vi "Get Ctl Value.vi"(8 "error in (no error)":errorcluster, 10 "Control Refs":refnum<vi>[](array[refnum]), 11 "Part in":refnum<class "Part.lvclass">) -> (0 "error out":errorcluster, 3 "Part out":refnum<class "Part.lvclass">)   [LabVIEW 2015, in "Part.lvclass"]
uses:
  Part.lvclass
  Part.lvclass/Part.ctl
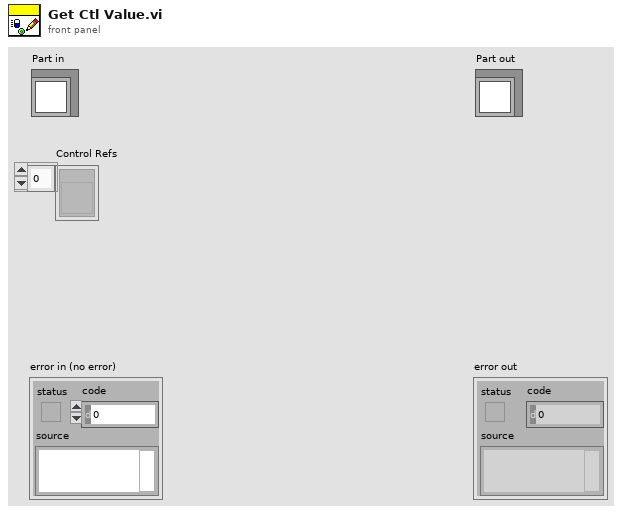
[diagram p1: front panel]
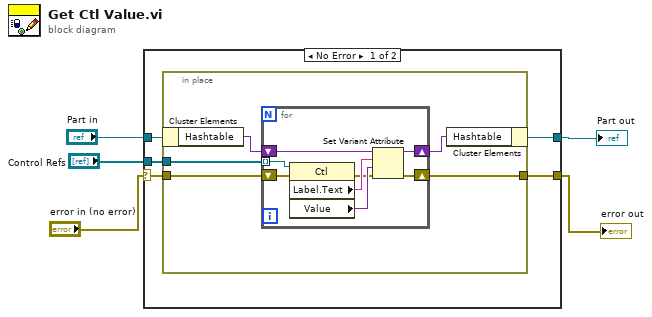
[diagram p0: block diagram]
diagram:
  n1 = case shown="No Error" "error in (no error)" {
    selector: "error in (no error)" -> [w8 w25]
    tunnel: [w7 w25] -> w4
    tunnel: [w6 w24] -> w2
    tunnel: "Part in" -> [w10 w24]
    tunnel: "Control Refs" -> [w9 _]
    frame No Error {
      n2 = in-place {
        in-place-border: w9 -> [w15]
        in-place-border: w8 -> [w14]
        in-place-border: [w11] -> w7
        n3 = in-place-cluster #1(w10) -> ("Hashtable"=w13:variant)
        n4 = for {
          tunnel: w15 -> [w23] mode=indexing
          shift-right: [w17] -> w12
          shift-left: w13 -> [w21]
          shift-right: [w16] -> w11
          shift-left: w14 -> [w22]
          n5 = property class="Ctl"(reference=w23, error in=w22) -> (error out=w18:errorcluster, "Label.Text"=w20:string, "Value"=w19:variant)  [unwired: 1 out]
          n6 = Set Variant Attribute(Variant=w21, name=w20, value=w19, error in=w18) -> (Variant out=w17:variant, error out=w16:errorcluster)  [unwired: 1 out]
        }
        n7 = in-place-cluster #1("Hashtable"=w12) -> (w6:refnum<class "Part.lvclass">)
      }
    }
    frame Error {
    }
  }
  "error out" <- w4
  "Part out" <- w2
